vi "Uninstall.vi"   [LabVIEW 2012, in "nisyscfg.lvlib"]
doc: "Uninstalls or installs software from a specified system. This VI does not remove files that were created on the target. Use the Format VI to reformat the target."
uses:
  <vilib>/nisyscfg/nisyscfg.lvlib
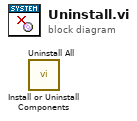
[diagram p0: block diagram]
diagram:
  n1 = call <vilib>:"Install or Uninstall Components.vi"() -> ()  [unwired: 9 in, 3 out]
  n2 = call <vilib>:"Uninstall All.vi"() -> ()  [unwired: 10 in, 2 out]
